vi "SGSA_Sweep_Only.vi"() -> ()   [LabVIEW 2023, in "SG_SA.lvlib"]
uses:
  SG_SA.lvlib
panel:
  in  "Air_Loss":dbl=8.0
  in  "Cable_Loss":dbl=8.0
  in  "Waiting Time(ms)":u32=1000
  in  "FileNote":string
  out "SG Power":i32
  in  "Stop Power":i32=8
  in  "Start Power":i32=-40
  in  "SG":refnum<visa-resource-name>="TCPIP0::192.168.100.200::inst0::INSTR"
  in  "AvgTimes":i32=5
  in  "SA":refnum<visa-resource-name>="TCPIP0::192.168.100.230::inst0::INSTR"
  out "Spectrum Data":cluster{"X":dbl, "Y":dbl}[](graph)
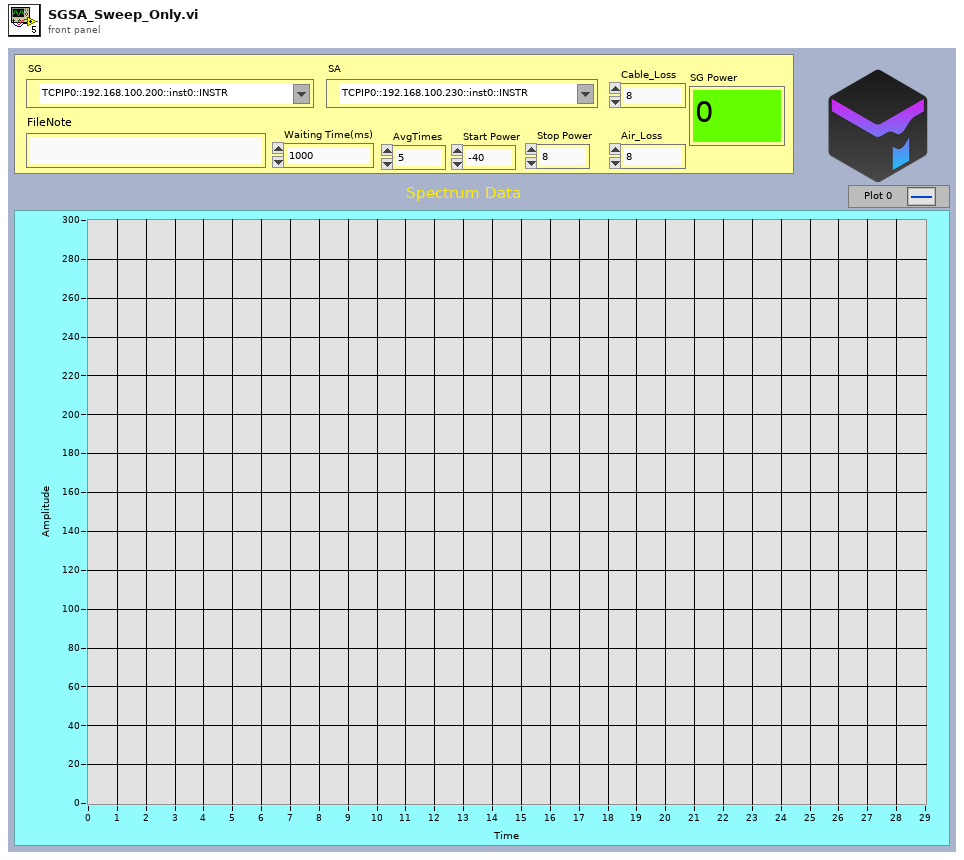
[diagram p1: front panel]
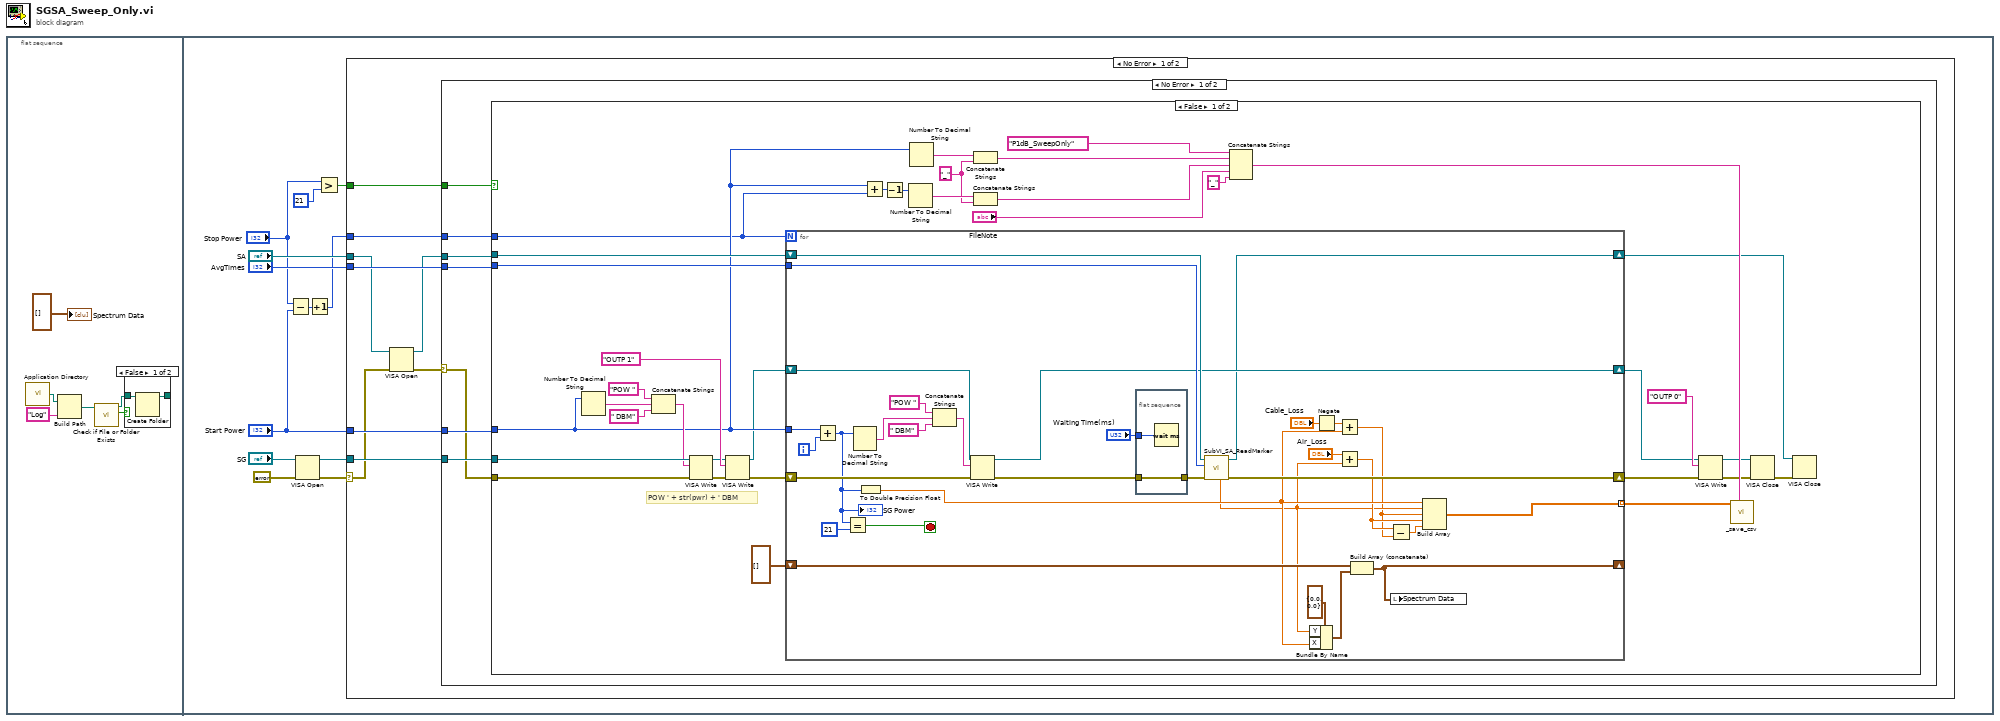
[diagram p0: block diagram]
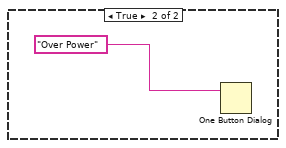
[diagram p3: hidden frame]
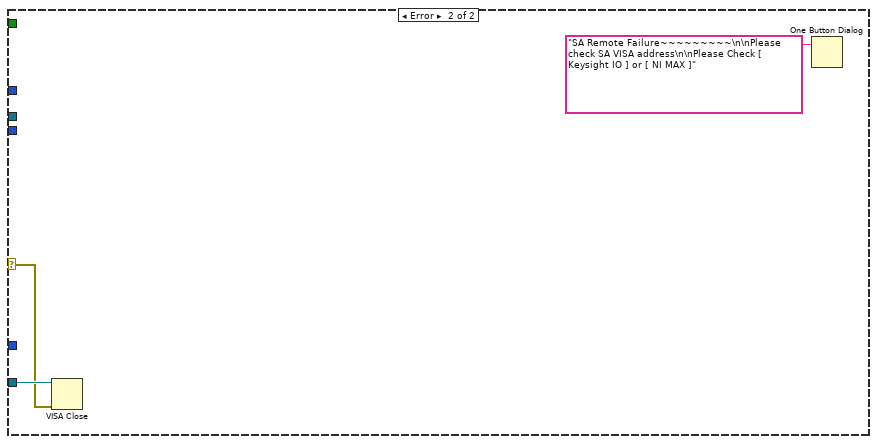
[diagram p4: hidden frame]
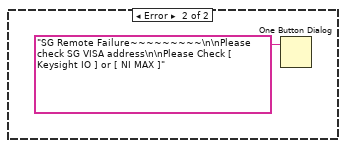
[diagram p5: hidden frame]
diagram:
  n1 = flat-sequence {
    frame #0 {
      n2 = call <vilib>:"Application Directory.vi"() -> ("Application Directory"=w5:path)
      n3 = Build Path(base path=w5, name or relative path="Log") -> (appended path=w2:path)
      n4 = call <vilib>:"Check if File or Folder Exists.vi"("path"=w2) -> ("file or folder exists?"=w4:bool, "dup path"=w3:path)  [unwired: 8 in, 1 out]
      n5 = case shown="False" w4 {
        tunnel: w3 -> [w8 w9]
        tunnel: [w7 w9] -> _
        frame False {
          n6 = Create Folder(path (use dialog)=w8) -> (created path=w7:path)  [unwired: 2 in, 2 out]
        }
        frame True {
        }
      }
      "Spectrum Data" <- cluster{"X":dbl, "Y":dbl}[] [] ("XY Graph")
    }
    frame #1 {
      n7 = Subtract(x="Stop Power", y="Start Power") -> (x-y=w17:i32)
      n8 = VISA Open(error in (no error)=errorcluster {"status"=FALSE, "code"=0, "source"=""}, VISA resource name="SG") -> (VISA resource name=w11:refnum<visa-resource-name>, error out=w10:errorcluster)  [unwired: 3 in]
      n9 = Increment(x=w17) -> (x+1=w16:i32)
      n10 = Greater?(x="Stop Power", y=21) -> (0:w20:bool)
      n11 = case shown="No Error" w10 {
        selector: w10 -> [w25 _]
        tunnel: "SA" -> [w23 _]
        tunnel: w20 -> [w30 _]
        tunnel: "Start Power" -> [w29 _]
        tunnel: "AvgTimes" -> [w28 _]
        tunnel: w16 -> [w27 _]
        tunnel: w11 -> [w26 _]
        frame No Error {
          n12 = VISA Open(error in (no error)=w25, VISA resource name=w23) -> (VISA resource name=w22:refnum<visa-resource-name>, error out=w24:errorcluster)  [unwired: 3 in]
          n13 = case shown="No Error" w24 {
            selector: w24 -> [w31 w108]
            tunnel: w22 -> [w37 _]
            tunnel: w30 -> [w36 _]
            tunnel: w29 -> [w35 _]
            tunnel: w28 -> [w34 _]
            tunnel: w27 -> [w33 _]
            tunnel: w26 -> [w32 w109]
            frame No Error {
              n14 = case shown="False" w36 {
                tunnel: w37 -> [w72 _]
                tunnel: w34 -> [w71 _]
                tunnel: w35 -> [w49 _]
                tunnel: w31 -> [w53 _]
                tunnel: w32 -> [w52 _]
                tunnel: w33 -> [w48 _]
                frame False {
                  w62 = "_"
                  # "POW ' + str(pwr) + ' DBM"
                  n15 = Number To Decimal String(number=w49) -> (decimal integer string=w55:string)  [unwired: 1 in]
                  n16 = Concatenate Strings("POW ", w55, " DBM") -> (w50:string)
                  n17 = VISA Write(VISA resource name=w52, write buffer=w50, error in (no error)=w53) -> (VISA resource name out=w51:refnum<visa-resource-name>, error out=w54:errorcluster)  [unwired: 1 out]
                  n18 = VISA Write(VISA resource name=w51, write buffer="OUTP 1", error in (no error)=w54) -> (VISA resource name out=w47:refnum<visa-resource-name>, error out=w70:errorcluster)  [unwired: 1 out]
                  n19 = for {
                    N: w48 -> [_]
                    tunnel: w71 -> [w103]
                    tunnel: w49 -> [w100]
                    shift-right: [w90] -> w67
                    shift-left: w70 -> [w102]
                    shift-right: [w92] -> w46
                    shift-left: w47 -> [w91]
                    tunnel: [w86] -> w43 mode=indexing
                    shift-right: [w85] -> w38
                    shift-left: w72 -> [w104]
                    shift-right: [w81] -> _
                    shift-left: cluster{"X":dbl, "Y":dbl}[] [] ("XY Graph") -> [w83]
                    i -> [w101]
                    stop <- w93 stop-if-true
                    n20 = Add(x=w100, y=w101) -> (x+y=w95:i32)
                    "SG Power" <- w95
                    n21 = Equal?(x=w95, y=21) -> (x = y?=w93:bool)
                    n22 = Number To Decimal String(number=w95) -> (decimal integer string=w97:string)  [unwired: 1 in]
                    n23 = To Double Precision Float(number=w95) -> (double precision float=w79:dbl)
                    n24 = Concatenate Strings("POW ", w97, " DBM") -> (w96:string)
                    n25 = VISA Write(VISA resource name=w91, write buffer=w96, error in (no error)=w102) -> (VISA resource name out=w92:refnum<visa-resource-name>, error out=w89:errorcluster)  [unwired: 1 out]
                    n26 = flat-sequence {
                      tunnel: w89 -> [w106]
                      tunnel: [w106] -> w88
                      tunnel: "Waiting Time(ms)" -> [w105]
                      frame #0 {
                        n27 = Wait (ms)(milliseconds to wait=w105) -> ()  [unwired: 1 out]
                      }
                    }
                    n28 = call "SubVI_SA_ReadMarker.vi"("error in (no error)"=w88, "AvgTimes"=w103, "VISA resource name"=w104) -> ("error out"=w90:errorcluster, "VISA resource name out"=w85:refnum<visa-resource-name>, "Marker Power"=w76:dbl)  [unwired: 5 in, 1 out]
                    n29 = Bundle By Name(cluster=cluster{"X":dbl, "Y":dbl} {"X"=0.0, "Y"=0.0} ("element"), "Y"=w76, "X"=w79) -> (w82:cluster{"X":dbl, "Y":dbl})
                    n30 = Negate(x="Cable_Loss") -> (-x=w73:dbl)
                    n31 = Add(x=w73, y=w79) -> (x+y=w75:dbl)
                    n32 = Add(x="Air_Loss", y=w76) -> (x+y=w77:dbl)
                    n33 = Build Array (concatenate)(w83, w82) -> (w81:cluster{"X":dbl, "Y":dbl}[])
                    n34 = Subtract(x=w77, y=w75) -> (x-y=w74:dbl)
                    n35 = local write "Spectrum Data"(w81) -> ()
                    n36 = Build Array(w79, w76, w75, w77, w74) -> (w86:dbl[])
                  }
                  n37 = Add(x=w49, y=w48) -> (x+y=w66:i32)
                  n38 = Decrement(x=w66) -> (x-1=w65:i32)
                  n39 = Number To Decimal String(number=w65) -> (decimal integer string=w63:string)  [unwired: 1 in]
                  n40 = Number To Decimal String(number=w49) -> (decimal integer string=w64:string)  [unwired: 1 in]
                  n41 = Concatenate Strings(w64, w62) -> (w60:string)
                  n42 = Concatenate Strings(w63, w62) -> (w59:string)
                  n43 = Concatenate Strings("P1dB_SweepOnly" ("delimiter (\\t)"), w60, w59, "FileNote", "_") -> (w58:string)
                  n44 = VISA Write(VISA resource name=w46, write buffer="OUTP 0", error in (no error)=w67) -> (VISA resource name out=w40:refnum<visa-resource-name>, error out=w41:errorcluster)  [unwired: 1 out]
                  n45 = call "_save_csv.vi"("delimiter (\\t)"=w58, "Data"=w43) -> ()  [unwired: 9 in, 1 out]
                  n46 = VISA Close(VISA resource name=w40, error in (no error)=w41) -> (error out=w39:errorcluster)
                  n47 = VISA Close(VISA resource name=w38, error in (no error)=w39) -> ()  [unwired: 1 out]
                }
                frame True {
                  n48 = One Button Dialog(message="Over Power") -> ()  [unwired: 1 in, 1 out]
                }
              }
            }
            frame Error {
              n49 = VISA Close(VISA resource name=w109, error in (no error)=w108) -> ()  [unwired: 1 out]
              n50 = One Button Dialog(message="SA Remote Failure~~~~~~~~~\n\nPlease check SA VISA address\n\nPlease Check [ Keysight IO ] or [ NI MAX ]") -> ()  [unwired: 1 in, 1 out]
            }
          }
        }
        frame Error {
          n51 = One Button Dialog(message="SG Remote Failure~~~~~~~~~\n\nPlease check SG VISA address\n\nPlease Check [ Keysight IO ] or [ NI MAX ]") -> ()  [unwired: 1 in, 1 out]
        }
      }
    }
  }
